vi "zdffgsdghbst.vi"() -> ()   [LabVIEW 2016]
uses:
  <vilib>/Platform/TimedLoop/XDataNode/timing_clust.ctl
  <vilib>/Platform/TimedLoop/XDataNode/nitl_modes.ctl
  <vilib>/Platform/TimedLoop/XDataNode/wakeup.ctl
  RT/sdfgserhgs.lvsc/StatechartState.ctl
  RT/sdfgserhgs.lvsc/State.ctl
  RT/sdfgserhgs.lvsc/CompanionDiagram.vi/1/SC Main.vi
  RT/sdfgserhgs.lvsc/CompanionDiagram.vi/1/Upd State.vi
  RT/sdfgserhgs.lvsc/CompanionDiagram.vi/1/Trans Graph0.vi
  RT/sdfgserhgs.lvsc/CompanionDiagram.vi/1/EnterGraphCore.vi
  RT/sdfgserhgs.lvsc/CompanionDiagram.vi
  <vilib>/Platform/TimedLoop/XDataNode/XDataNode.xnode
  RT/sdfgserhgs.lvsc/Inputs.ctl
  RT/sdfgserhgs.lvsc/Trigger.ctl
  <vilib>/Statechart/Infrastructure/RTStatechart/RunTime SCN.xnode
  RT/sdfgserhgs.lvsc
  RT/sdfgserhgs.lvsc/Outputs.ctl
  <vilib>/Platform/TimedLoop/XDataNode/XDNodeRunTimeDep.lvlib
panel:
  out "Error":errorcluster
  out "Diagram Display":picture
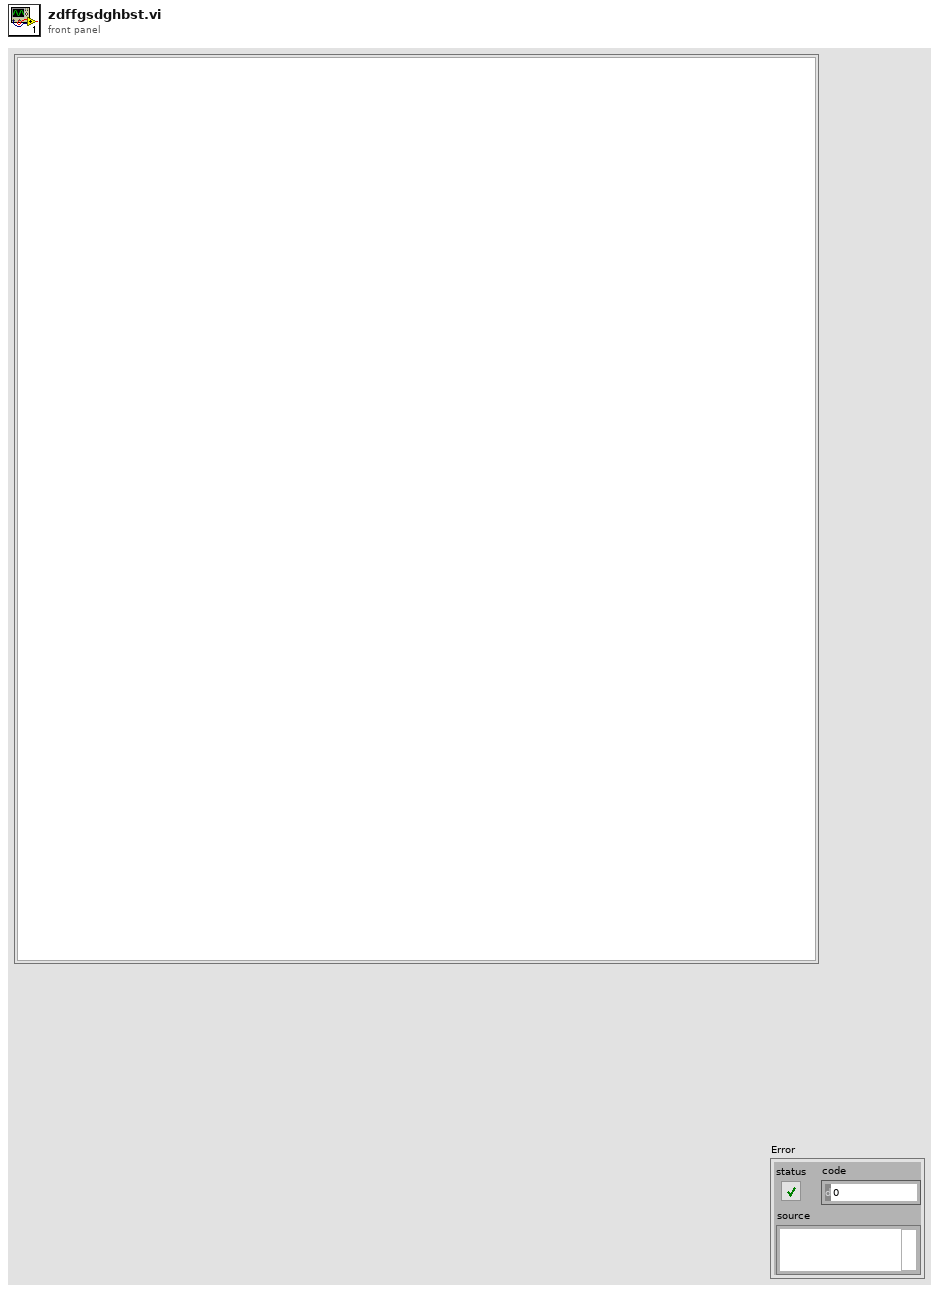
[diagram p1: front panel]
types:
  T1 = typedef "XDNodeRunTimeDep.lvlib/timing_clust.ctl" = cluster{"Expected End [f-1]":u64, "Actual End [f-1]":u64, "Finished Late? [f-1]":bool, "Expected End [i-1]":u64, "Actual End [i-1]":u64, "Finished Late? [i-1]":bool, "Expected Start [i]":u64, "Actual Start [i]":u64, "Expected Start [f]":u64, "Actual Start [f]":u64, "Source Name":string, "Structure Name":string, "Period":i64, "Deadline":i64, "Offset":i64, "Start":i64, "Priority":i32, "Timeout":i32, "Mode":T2, "Wakeup Reason":T3, "Error":errorcluster, "Source Type":string, "Secondary Source Type":string, "Global End Time":u64, "Global Start Time":u64, "Frame Duration":u64, "Iteration Duration":u64, "Assigned CPU":i32, "I/O Scan Engine Mode":u32}
  T2 = typedef "XDNodeRunTimeDep.lvlib/nitl_modes.ctl" = enum32{"No Change", "Process missed periods, maintain original phase", "Discard missed periods, maintain original phase", "Process missed periods, ignore original phase", "Discard missed periods, ignore original phase"}
  T3 = typedef "XDNodeRunTimeDep.lvlib/wakeup.ctl" = enum32{"Normal", "Aborted", "Asynchronous wakeup", "Timing source error", "Timed loop error", "Timeout"}
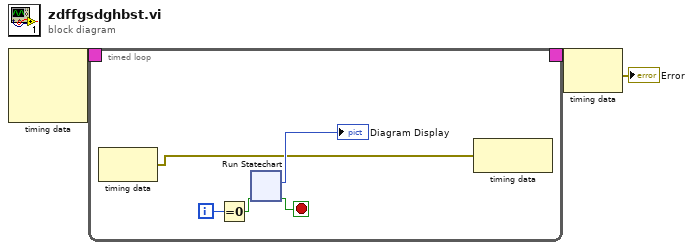
[diagram p0: block diagram]
diagram:
  n1 = node-c288() -> (w3:T1)  [unwired: 3 in]
  n2 = timed-loop {
    timing: w3 -> [_]
    timing-out: [_] -> w2
    i -> [w5]
    stop <- w4 stop-if-true
    n3 = node-c288() -> (w7:errorcluster)  [unwired: 1 in]
    n4 = Equal To 0?(x=w5) -> (x = 0?=w6:bool)
    n5 = xnode "Run Statechart"("Init?"=w6) -> ("Terminated?"=w4:bool, "Diagram Display"=→"Diagram Display":picture)  [unwired: 3 in, 2 out]
    n6 = node-c288(w7) -> ()  [unwired: 1 out]
  }
  n7 = node-c288(w2) -> (→"Error":errorcluster)
